vi "Control Panel Values Changed.vi"(8 "error in (no error)":errorcluster, 9 "Old value":variant, 10 "New value":variant, 11 "LakeShore 340 in":refnum<class "LakeShore 340.lvclass">) -> (0 "error out":errorcluster, 3 "LakeShore 340 out":refnum<class "LakeShore 340.lvclass">)   [LabVIEW 2015, in "LakeShore 340.lvclass"]
uses:
  LakeShore 340.lvclass
  LakeShore340 Front Panel Data.ctl
  LakeShore340 Heater Ranges.ctl
  Neocera/Neocera Set Point Aproach.ctl
  Instrument/Read VISA Resource.vi
  Instrument/Write VISA Resource.vi
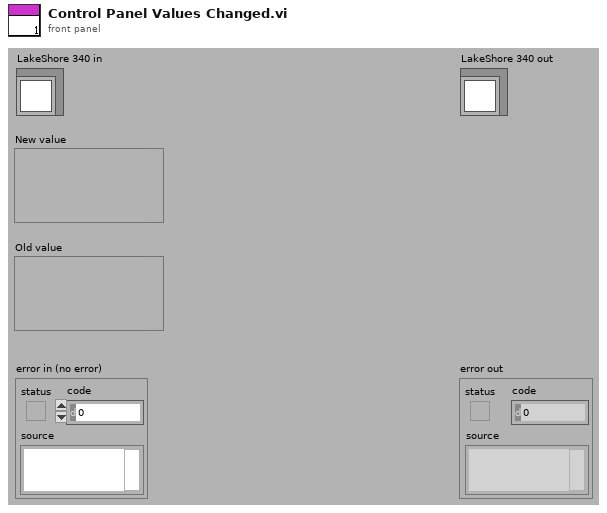
[diagram p1: front panel]
types:
  T1 = typedef "LakeShore340 Front Panel Data.ctl" = cluster{"Record heater":bool, "A":bool, "B":bool, "Record RAW":bool, "Set point":dbl, "Set Heater Range":T2, "Approach":T3, "Ramp rate, K/min":dbl, "C":bool, "D":bool}
  T2 = typedef "LakeShore340 Heater Ranges.ctl" = enum16{"0 (Off)", "1 (5 mW)", "2 (50 mW)", "3 (500 mW)", "4 (5 W)", "5 (50 W)"}
  T3 = typedef "Neocera Set Point Aproach.ctl" = enum16{"Instant", "Ramp"}
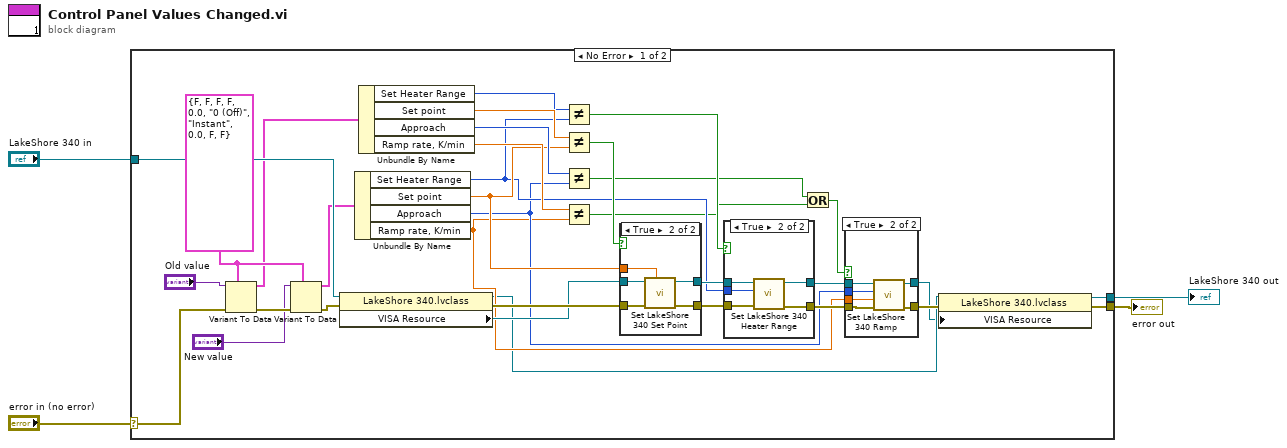
[diagram p0: block diagram]
diagram:
  n1 = case shown="No Error" "error in (no error)" {
    selector: "error in (no error)" -> [w31 w61]
    tunnel: [w6 w61] -> w3
    tunnel: [w7 w60] -> w1
    tunnel: "LakeShore 340 in" -> [w35 w60]
    frame No Error {
      w32 = T1 {"Record heater"=FALSE, "A"=FALSE, "B"=FALSE, "Record RAW"=FALSE, "Set point"=0.0, "Set Heater Range"=enum."0 (Off)", "Approach"=enum."Instant", "Ramp rate, K/min"=0.0, "C"=FALSE, "D"=FALSE} ("Data")
      n2 = Variant To Data(error in=w31, type=w32, Variant="Old value") -> (data=w26:T1, error out=w37:errorcluster)
      n3 = Variant To Data(error in=w37, type=w32, Variant="New value") -> (data=w25:T1, error out=w36:errorcluster)
      n4 = property class="LakeShore 340.lvclass"(reference=w35, error in=w36) -> (reference out=w8:refnum<class "LakeShore 340.lvclass">, error out=w24:errorcluster, "VISA Resource"=w23:refnum<visa-resource-name>)
      n5 = Unbundle By Name(w25) -> ("Set Heater Range"=w18:T2, "Set point"=w21:dbl, "Approach"=w11:T3, "Ramp rate, K/min"=w10:dbl)
      n6 = Unbundle By Name(w26) -> ("Set Heater Range"=w29:T2, "Set point"=w30:dbl, "Approach"=w28:T3, "Ramp rate, K/min"=w27:dbl)
      n7 = Not Equal?(x=w29, y=w18) -> (x != y?=w17:bool)
      n8 = Not Equal?(x=w30, y=w21) -> (x != y?=w22:bool)
      n9 = Not Equal?(x=w28, y=w11) -> (x != y?=w15:bool)
      n10 = Not Equal?(x=w27, y=w10) -> (x != y?=w14:bool)
      n11 = case shown="True" w22 {
        tunnel: w24 -> [w54 w59]
        tunnel: w23 -> [w53 w58]
        tunnel: w21 -> [_ w57]
        tunnel: [w54 w56] -> w20
        tunnel: [w53 w55] -> w19
        frame False {
        }
        frame True {
          n12 = call "Set LakeShore 340 Set Point.vi"("Set point"=w57, "error in (no error)"=w59, "VISA Resource Name"=w58) -> ("error out"=w56:errorcluster, "VISA Resource Name Out"=w55:refnum<visa-resource-name>)  [unwired: 7 in]
        }
      }
      n13 = case shown="True" w17 {
        tunnel: w20 -> [w47 w52]
        tunnel: w19 -> [w46 w51]
        tunnel: w18 -> [_ w50]
        tunnel: [w46 w49] -> w12
        tunnel: [w47 w48] -> w16
        frame False {
        }
        frame True {
          n14 = call "Set LakeShore 340 Heater Range.vi"("error in (no error)"=w52, "Set Heater Range"=w50, "VISA resource name"=w51) -> ("error out"=w48:errorcluster, "VISA resource name out"=w49:refnum<visa-resource-name>)  [unwired: 7 in]
        }
      }
      n15 = Or(x=w15, y=w14) -> (x .or. y?=w13:bool)
      n16 = case shown="True" w13 {
        tunnel: w16 -> [w39 w45]
        tunnel: w12 -> [w38 w44]
        tunnel: [w39 w42] -> w9
        tunnel: [w38 w43] -> w5
        tunnel: w11 -> [_ w41]
        tunnel: w10 -> [_ w40]
        frame False {
        }
        frame True {
          n17 = call "Set LakeShore 340 Ramp.vi"("error in (no error)"=w45, "Ramp rate, K/min"=w40, "Approach"=w41, "VISA resource name"=w44) -> ("error out"=w42:errorcluster, "VISA resource name out"=w43:refnum<visa-resource-name>)  [unwired: 6 in]
        }
      }
      n18 = property class="LakeShore 340.lvclass"(reference=w8, error in=w9, "VISA Resource"=w5) -> (reference out=w7:refnum<class "LakeShore 340.lvclass">, error out=w6:errorcluster)
    }
    frame Error {
    }
  }
  "error out" <- w3
  "LakeShore 340 out" <- w1
